vi "Forebrain_checkoffMissions.vi"(10 "MissionArray in":refnum<class "GenericMission.lvclass">[](array[class]), 11 "Waypoints":refnum<queue>) -> (1 "new Mission?":bool, 2 "MissionArray out":refnum<class "GenericMission.lvclass">[](array[class]), 3 "Waypoints out":refnum<queue>)   [LabVIEW 2013]
doc: "When there is only one waypoint left in the queue, drop the mission from the queue.\nAlso removes mission from mission queue\n\nKaitlin (4/16)"
uses:
  Classes/Waypoint/Waypoint.lvclass
  Classes/Missions/GenericMission/GenericMission.lvclass
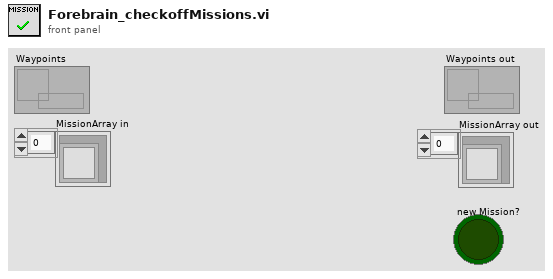
[diagram p1: front panel]
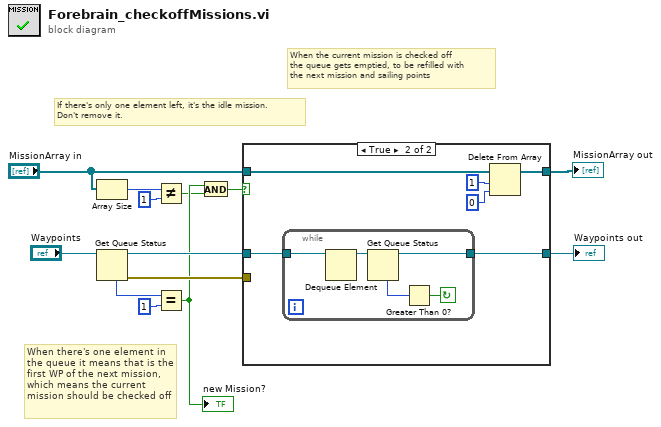
[diagram p0: block diagram]
diagram:
  # "When the current mission is checked off\nthe queue gets emptied, to be refilled with\nthe next mission and sailing points"
  # "If there's only one element left, it's the idle mission.\nDon't remove it."
  # "When there's one element in the queue it means that is the first WP of the next mission, which means the current mission should be checked off"
  n1 = Array Size(array="MissionArray in") -> (size(s)=w5:i32)
  n2 = Get Queue Status(queue="Waypoints") -> (queue out=w12:refnum<queue>, error out=w11:errorcluster, # elements in queue=w8:i32)  [unwired: 2 in, 5 out]
  n3 = Not Equal?(x=w5, y=1) -> (x != y?=w1:bool)
  n4 = Equal?(x=w8, y=1) -> (x = y?=w3:bool)
  "new Mission?" <- w3
  n5 = And(x=w3, y=w1) -> (x .and. y?=w2:bool)
  n6 = case shown="True" w2 {
    tunnel: w12 -> [w15 w17]
    tunnel: w11 -> [_ _]
    tunnel: [w15 w16] -> w10
    tunnel: "MissionArray in" -> [w14 w21]
    tunnel: [w14 w20] -> w9
    frame False {
    }
    frame True {
      n7 = while {
        tunnel: w17 -> [w24]
        tunnel: [w23] -> w16
        stop <- w26 continue-if-true
        n8 = Dequeue Element(queue=w24) -> (queue out=w22:refnum<queue>)  [unwired: 2 in, 3 out]
        n9 = Get Queue Status(queue=w22) -> (queue out=w23:refnum<queue>, # elements in queue=w25:i32)  [unwired: 2 in, 6 out]
        n10 = Greater Than 0?(x=w25) -> (x > 0?=w26:bool)
      }
      n11 = Delete From Array(array=w21, length=1, index=0) -> (array with subset deleted=w20:refnum<class "GenericMission.lvclass">[])  [unwired: 1 out]
    }
  }
  "Waypoints out" <- w10
  "MissionArray out" <- w9
